vi "2.vi"() -> ()   [LabVIEW 2015]
panel:
  out "Updated Duplicated Points":i32
  out "Update Missing Points":i32
  in  "Current Missing Points":i32
  in  "Previous Producer Iterations":i32
  in  "Producer Iterations":i32
  in  "Current Duplicated Points":i32
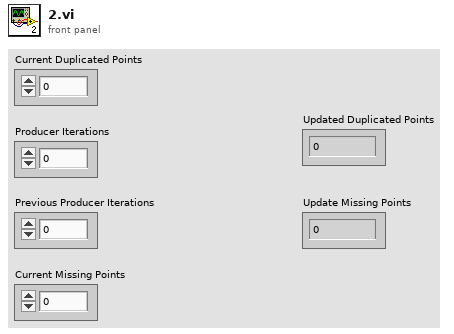
[diagram p1: front panel]
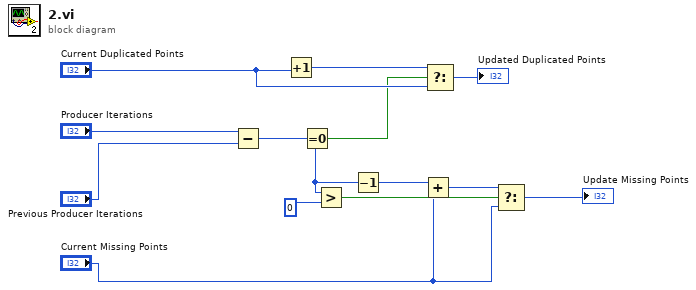
[diagram p0: block diagram]
diagram:
  n1 = Subtract(x="Producer Iterations", y="Previous Producer Iterations") -> (x-y=w8:i32)
  n2 = Increment(x="Current Duplicated Points") -> (x+1=w13:i32)
  n3 = Equal To 0?(x=w8) -> (x = 0?=w9:bool)
  n4 = Greater?(x=w8, y=0) -> (0:w5:bool)
  n5 = Decrement(x=w8) -> (x-1=w6:i32)
  n6 = Add(x=w6, y="Current Missing Points") -> (x+y=w4:i32)
  n7 = Select(t=w13, s=w9, f="Current Duplicated Points") -> (s? t:f=→"Updated Duplicated Points":i32)
  n8 = Select(t=w4, s=w5, f="Current Missing Points") -> (s? t:f=→"Update Missing Points":i32)
